vi "ELVIS III v1.0 Build MUX Configuration AO Continuous.vi"(11 "AO (Continuous) Channels List":T1 caption="AI (N Samples) Channels List") -> (3 "Channel Reservation Info":T3)   [LabVIEW 2021]
uses:
  <vilib>/myRIO/Common/Instrument Driver Framework/ELVIS III v1.0/Resource Manager/typedefs/ELVIS III v1.0 Channel Reservation List.ctl
  <vilib>/myRIO/Common/Instrument Driver Framework/ELVIS III v1.0/Resource Manager/typedefs/ELVIS III v1.0 Channel Reservation Info.ctl
  <vilib>/myRIO/Common/Instrument Driver Framework/ELVIS III v1.0/Resource Manager/typedefs/ELVIS III v1.0 Connector List.ctl
  <vilib>/myRIO/Common/Instrument Driver Framework/ELVIS III v1.0/AO Continuous/typedefs/AO Continuous Channels List.ctl
  <vilib>/myRIO/Common/Instrument Driver Framework/ELVIS III v1.0/AO Continuous/typedefs/ELVIS III v1.0 AO Continuous Channels Enum.ctl
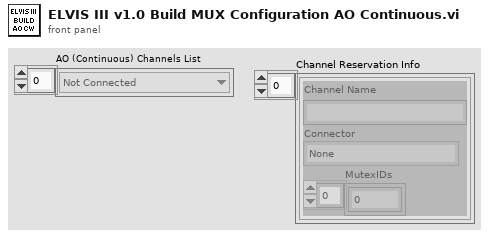
[diagram p1: front panel]
types:
  T1 = typedef "AO Continuous Channels List.ctl" = T2[]
  T2 = typedef "ELVIS III v1.0 AO Continuous Channels Enum.ctl" = enum16{"Not Connected", "A/AO0 (Continuous)", "A/AO1 (Continuous)", "B/AO0 (Continuous)", "B/AO1 (Continuous)"}
  T3 = typedef "ELVIS III v1.0 Channel Reservation List.ctl" = T4[]
  T4 = typedef "ELVIS III v1.0 Channel Reservation Info.ctl" = cluster{"Channel Name":string, "Connector":T5, "MutexIDs":u32[]}
  T5 = typedef "ELVIS III v1.0 Connector List.ctl" = enum32{"None", "ConnectorA", "ConnectorB"}
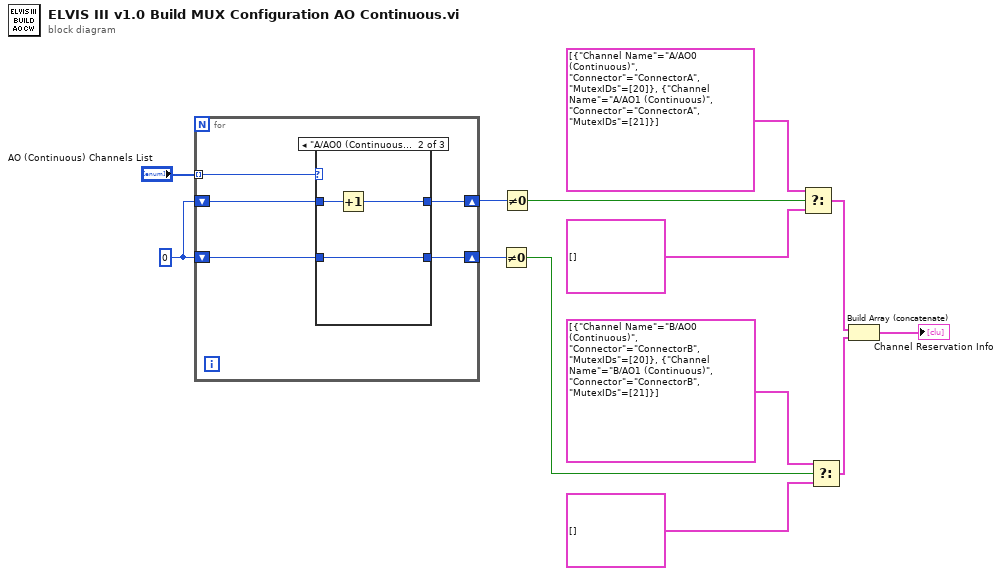
[diagram p0: block diagram]
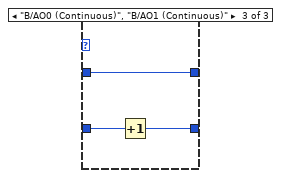
[diagram p3: hidden frame]
diagram:
  w6 = u8 0
  n1 = for {
    tunnel: "AO (Continuous) Channels List" -> [w18] mode=indexing
    shift-right: [w16] -> w3
    shift-left: w6 -> [w17]
    shift-right: [w14] -> w2
    shift-left: w6 -> [w15]
    n2 = case shown="\"A/AO0 (Continuous)\", \"A/AO1 (Continuous)\"" w18 {
      tunnel: w17 -> [w20 w22 w26]
      tunnel: [w20 w21 w26] -> w16
      tunnel: w15 -> [w19 w23 w25]
      tunnel: [w19 w23 w24] -> w14
      frame "Not Connected", Default {
      }
      frame "A/AO0 (Continuous)", "A/AO1 (Continuous)" {
        n3 = Increment(x=w22) -> (x+1=w21:u8)
      }
      frame "B/AO0 (Continuous)", "B/AO1 (Continuous)" {
        n4 = Increment(x=w25) -> (x+1=w24:u8)
      }
    }
  }
  n5 = Not Equal To 0?(x=w2) -> (x != 0?=w4:bool)
  n6 = Not Equal To 0?(x=w3) -> (x != 0?=w5:bool)
  n7 = Select(t=T4[] [{"Channel Name"="A/AO0 (Continuous)", "Connector"=enum."ConnectorA", "MutexIDs"=[20]}, {"Channel Name"="A/AO1 (Continuous)", "Connector"=enum."ConnectorA", "MutexIDs"=[21]}], s=w5, f=T4[] []) -> (s? t:f=w11:T4[])
  n8 = Select(t=T4[] [{"Channel Name"="B/AO0 (Continuous)", "Connector"=enum."ConnectorB", "MutexIDs"=[20]}, {"Channel Name"="B/AO1 (Continuous)", "Connector"=enum."ConnectorB", "MutexIDs"=[21]}], s=w4, f=T4[] []) -> (s? t:f=w8:T4[])
  n9 = Build Array (concatenate)(w11, w8) -> (→"Channel Reservation Info":T4[])
